vi "setValue.vi"(8 "error in (no error)":errorcluster, 9 "Value":variant, 10 "Key":string, 11 "HashMap in":refnum<class "HashMap.lvclass">) -> (0 "error out":errorcluster, 3 "HashMap out":refnum<class "HashMap.lvclass">)   [LabVIEW 2017, in "HashMap.lvclass"]
uses:
  <userlib>/836-Library/Data_Structures/HashMap/HashMap.lvclass
  <userlib>/836-Library/Data_Structures/HashMap/HashMap.lvclass/HashMap.ctl
  <vilib>/Utility/error.llb/Error Cluster From Error Code.vi
  <vilib>/ErrorRing/Error Ring.xnode
  <userlib>/836-Library/Data_Structures/Bucket/Bucket.lvclass
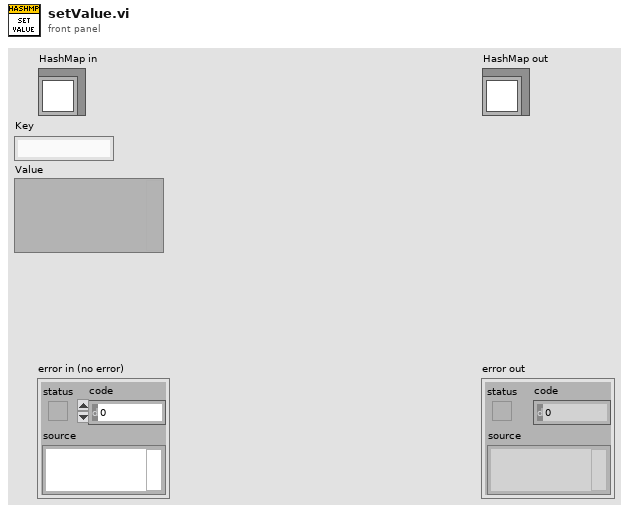
[diagram p1: front panel]
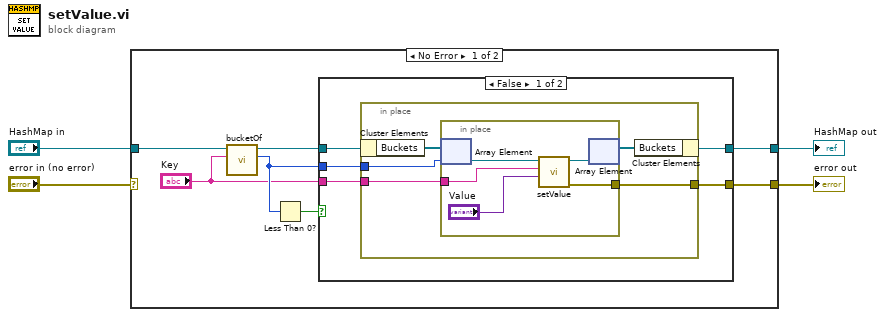
[diagram p0: block diagram]
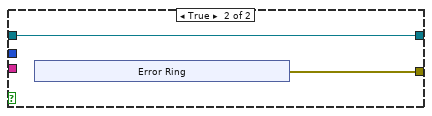
[diagram p2: hidden frame]
diagram:
  n1 = case shown="No Error" "error in (no error)" {
    selector: "error in (no error)" -> [_ w35]
    tunnel: [w6 w35] -> w3
    tunnel: [w5 w34] -> w1
    tunnel: "HashMap in" -> [w11 w34]
    frame No Error {
      n2 = call <userlib>:"bucketOf.vi"("Key"="Key", "HashMap in"=w11) -> ("Bucket Index"=w8:i32, "HashMap out"=w9:refnum<class "HashMap.lvclass">)  [unwired: 7 in, 1 out]
      n3 = Less Than 0?(x=w8) -> (x < 0?=w10:bool)
      n4 = case shown="False" w10 {
        tunnel: w9 -> [w16 w28]
        tunnel: w8 -> [w15 _]
        tunnel: "Key" -> [w14 _]
        tunnel: [w13 w27] -> w6
        tunnel: [w12 w28] -> w5
        frame False {
          n5 = in-place {
            in-place-border: w15 -> [w20]
            in-place-border: w14 -> [w19]
            in-place-border: [w18] -> w13
            n6 = in-place-cluster #1(w16) -> ("Buckets"=w21:refnum<class "Bucket.lvclass">[])
            n7 = in-place {
              in-place-border: w19 -> [w24]
              in-place-border: [w22] -> w18
              n8 = in-place-array #2(w21, w20) -> (w26:refnum<class "Bucket.lvclass">)
              n9 = call <userlib>:"setValue.vi"("Value"="Value", "Key"=w24, "Bucket in"=w26) -> ("error out"=w22:errorcluster, "Bucket out"=w25:refnum<class "Bucket.lvclass">)  [unwired: 7 in]
              n10 = in-place-array #2(w25) -> (w17:refnum<class "Bucket.lvclass">[])  [unwired: 1 out]
            }
            n11 = in-place-cluster #1("Buckets"=w17) -> (w12:refnum<class "HashMap.lvclass">)
          }
        }
        frame True {
          n12 = xnode "Error Ring"() -> ("error out"=w27:errorcluster)
        }
      }
    }
    frame Error {
    }
  }
  "error out" <- w3
  "HashMap out" <- w1
